vi "Base Ctrl Set Names.vi"() -> (4 "Base Names":T1, 15 "Canceled":bool)   [LabVIEW 2020]
uses:
  Base Ctrl Type Defs/Base Ctrl Setup Names.ctl
  <vilib>/Utility/miscctls.llb/LVPointTypeDef.ctl
panel:
  in  "Output Ports":string[](array[string])
  in  "Lamps":string[](array[string])
  in  "Turet Filter Names":string[](array[string])
  in  "Objecive Names":string[](array[string])
  in  "Cancel":bool
  in  "Save":bool
  # "1"
  # "1"
  # "2"
  # "2"
  # "3"
  # "3"
  # "4"
  # "4"
  # "5"
  # "5"
  # "6"
  # "6"
  # "1"
  # "1"
  # "2"
  # "2"
  # "3"
  # "3"
  # "4"
  # "4"
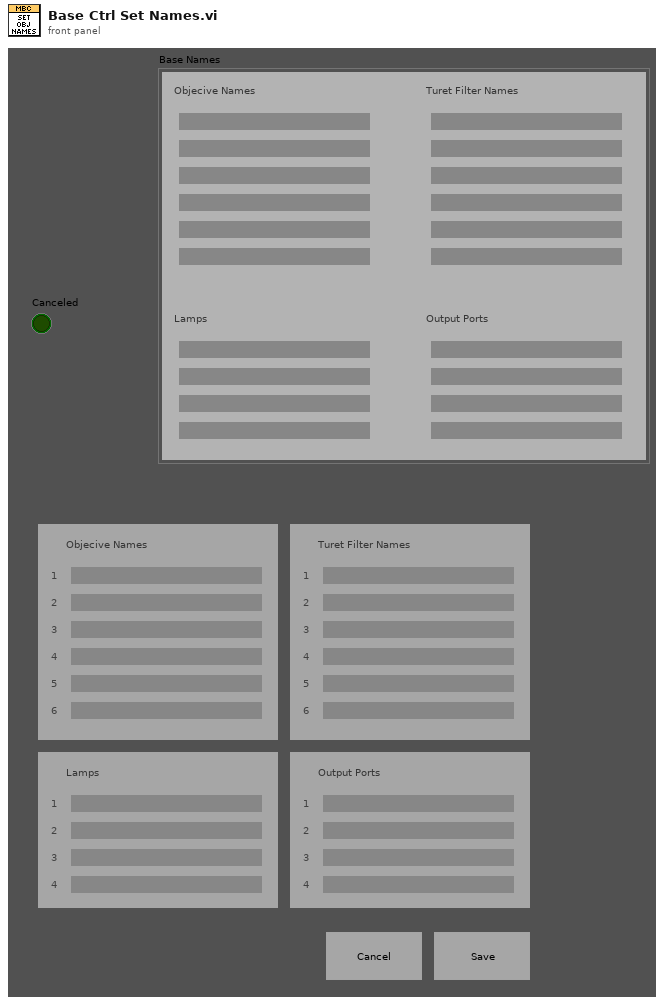
[diagram p1: front panel]
types:
  T1 = typedef "Base Ctrl Setup Names.ctl" = cluster{"Objecive Names":string[], "Turet Filter Names":string[], "Lamps":string[], "Output Ports":string[]}
  T2 = enum16{"Always On", "Always Off", "Off While Running"}
  T3 = typedef "LVPointTypeDef.ctl" = cluster{"Horizontal":i16, "Vertical":i16}
  T4 = typedef "LVBoundsTypeDef.ctl" = cluster{"Width":u32, "Height":u32}
  T5 = typedef "LVRectTypeDef.ctl" = cluster{"Left":i16, "Top":i16, "Right":i16, "Bottom":i16}
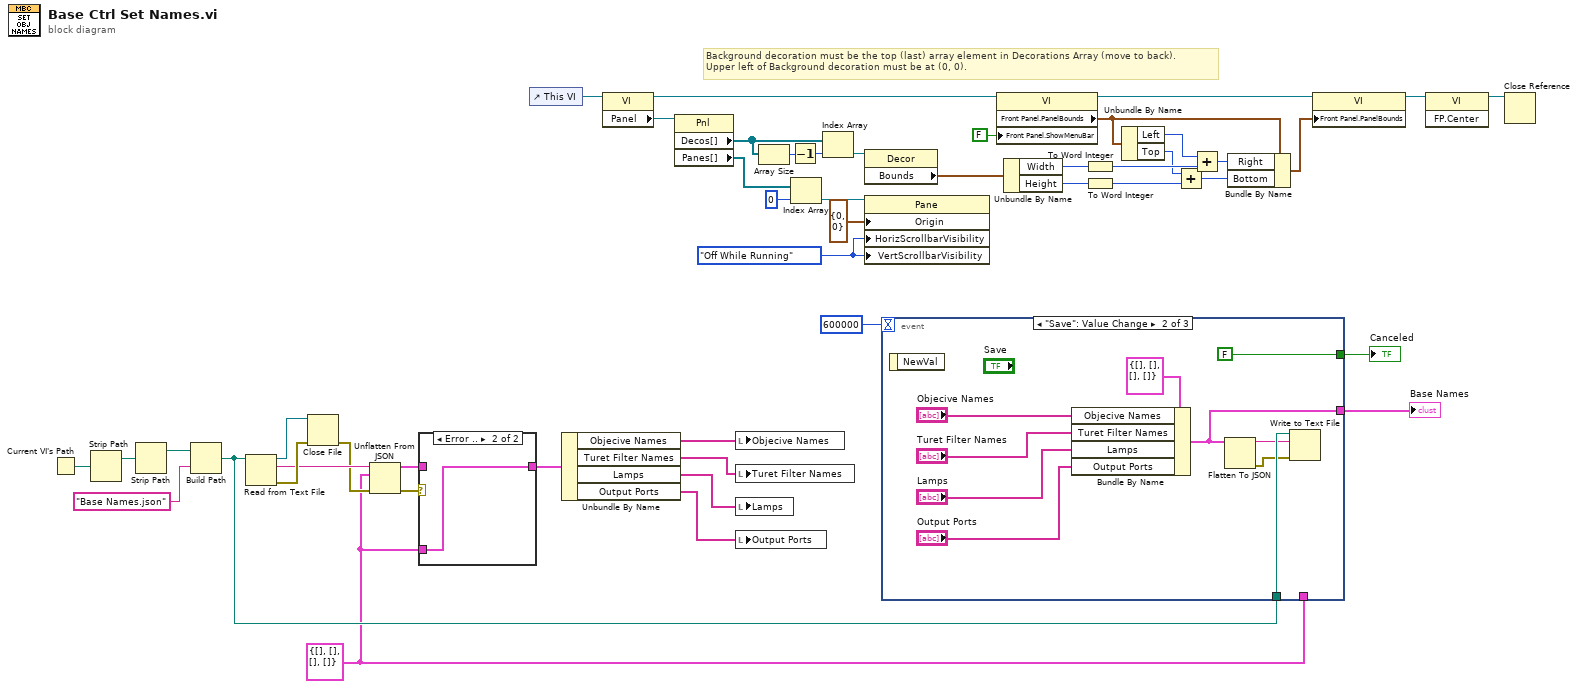
[diagram p0: block diagram]
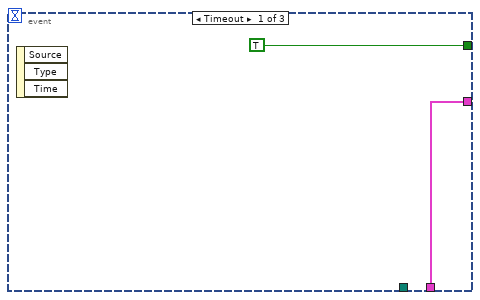
[diagram p3: hidden frame]
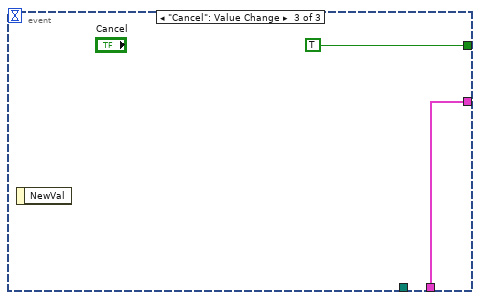
[diagram p4: hidden frame]
diagram:
  w7 = T1 {"Objecive Names"=[], "Turet Filter Names"=[], "Lamps"=[], "Output Ports"=[]} ("Base Names")
  w38 = T2."Off While Running" ("Vertical Scrollbar Visibility")
  # "Background decoration must be the top (last) array element in Decorations Array (move to back).\nUpper left of Background decoration must be at (0, 0)."
  n1 = Current VI's Path() -> (path=w10:path)
  n2 = Strip Path(path=w10) -> (stripped path=w9:path)  [unwired: 1 out]
  n3 = Strip Path(path=w9) -> (stripped path=w19:path)  [unwired: 1 out]
  n4 = Build Path(base path=w19, name or relative path="Base Names.json") -> (appended path=w8:path)
  n5 = Read from Text File(file (use dialog)=w8) -> (refnum out=w17:refnum<file>, text=w15:string, error out=w16:errorcluster)  [unwired: 3 in, 1 out]
  n6 = Close File(refnum=w17, error in=w16) -> (error out=w14:errorcluster)  [unwired: 1 out]
  n7 = Unflatten From JSON(JSON string=w15, type and defaults=w7, error in (no error)=w14) -> (value=w12:T1, error out=w13:errorcluster)  [unwired: 4 in]
  n8 = case shown="Error .." w13 {
    tunnel: w12 -> [w48 _]
    tunnel: [w48 w49] -> w6
    tunnel: w7 -> [_ w49]
    frame No Error {
    }
    frame Error {
    }
  }
  n9 = control-ref of="This VI"() -> (w24:refnum<vi>)
  n10 = Unbundle By Name(w6) -> ("Objecive Names"=w5:string[], "Turet Filter Names"=w4:string[], "Lamps"=w3:string[], "Output Ports"=w2:string[])
  n11 = property class="VI"(reference=w24) -> (reference out=w39:refnum<vi>, "Panel"=w32:refnum<vi>)  [unwired: 1 in, 1 out]
  n12 = property class="Pnl"(reference=w32) -> ("Decos[]"=w26:refnum<vi>[], "Panes[]"=w35:refnum<vi>[])  [unwired: 1 in, 2 out]
  n13 = local write "Objecive Names"(w5) -> ()
  n14 = local write "Turet Filter Names"(w4) -> ()
  n15 = local write "Lamps"(w3) -> ()
  n16 = local write "Output Ports"(w2) -> ()
  n17 = Array Size(array=w26) -> (size(s)=w31:i32)
  n18 = Decrement(x=w31) -> (x-1=w25:i32)
  n19 = Index Array(array=w35, index=0) -> (element=w34:refnum<vi>)
  n20 = Index Array(array=w26, index=w25) -> (element=w37:refnum<vi>)
  n21 = property class="Decor"(reference=w37) -> ("Bounds"=w40:T4)  [unwired: 1 in, 2 out]
  n22 = property class="Pane"(reference=w34, "Origin"=T3 {"Horizontal"=0, "Vertical"=0}, "HorizScrollbarVisibility"=w38, "VertScrollbarVisibility"=w38) -> ()  [unwired: 1 in, 2 out]
  n23 = event shown="[1] \"Save\": Value Change" {
    selector: _ -> [_ _ _]
    dyn-events: _ -> [_ _ _]
    timeout: 600000 -> [_ _ _]
    tunnel: w8 -> [_ w61 _]
    tunnel: [TRUE FALSE TRUE] -> w11
    tunnel: [w50 w56 w62] -> w1
    tunnel: w7 -> [w50 _ w62]
    event Timeout {
      n24 = event-data() -> ()  [unwired: 1 in, 3 out]
    }
    event "Save": Value Change {
      n25 = event-data() -> ()  [unwired: 1 in, 1 out]
      n26 = Bundle By Name(cluster=T1 {"Objecive Names"=[], "Turet Filter Names"=[], "Lamps"=[], "Output Ports"=[]} ("Base Names"), "Objecive Names"="Objecive Names", "Turet Filter Names"="Turet Filter Names", "Lamps"="Lamps", "Output Ports"="Output Ports") -> (w56:T1)
      n27 = Flatten To JSON(anything=w56) -> (JSON string=w60:string, 11:w59:errorcluster)  [unwired: 2 in]
      n28 = Write to Text File(file (use dialog)=w61, text=w60, error in=w59) -> ()  [unwired: 1 in, 3 out]
    }
    event "Cancel": Value Change {
      n29 = event-data() -> ()  [unwired: 1 in, 1 out]
    }
  }
  "Canceled" <- w11
  "Base Names" <- w1
  n30 = property class="VI"(reference=w39, "Front Panel.ShowMenuBar"=FALSE ("Front Panel Window:Show Menu Bar")) -> (reference out=w41:refnum<vi>, "Front Panel.PanelBounds"=w42:T5)  [unwired: 1 in, 1 out]
  n31 = Unbundle By Name(w40) -> ("Width"=w45:u32, "Height"=w47:u32)
  n32 = To Word Integer(number=w45) -> (16bit integer=w46:i16)
  n33 = To Word Integer(number=w47) -> (16bit integer=w27:i16)
  n34 = Unbundle By Name(w42) -> ("Left"=w44:i16, "Top"=w29:i16)
  n35 = Add(x=w29, y=w27) -> (x+y=w28:i16)
  n36 = Add(x=w44, y=w46) -> (x+y=w30:i16)
  n37 = Bundle By Name(cluster=w42, "Right"=w30, "Bottom"=w28) -> (w43:T5)
  n38 = property class="VI"(reference=w41, "Front Panel.PanelBounds"=w43) -> (reference out=w21:refnum<vi>)  [unwired: 1 in, 1 out]
  n39 = invoke class="VI" method="FP.Center"(reference=w21) -> (reference out=w23:refnum<vi>)  [unwired: 2 in, 2 out]
  n40 = Close Reference(reference=w23) -> ()  [unwired: 1 in, 1 out]
